vi "Adjust Focus.vi"(8 "error in":errorcluster, 10 "FocusPos":i64, 11 "Flir A700 in":refnum<class "Flir A700.lvclass">) -> (0 "error out":errorcluster, 3 "Flir A700 out":refnum<class "Flir A700.lvclass">)   [LabVIEW 2024, in "Flir A700.lvclass"]
uses:
  Flir A700.lvclass
  Flir A700.lvclass/Flir A700.ctl
  <resource>/objmgr/imaqdx.rc
  <vilib>/userDefined/High Color/IMAQdx.ctl
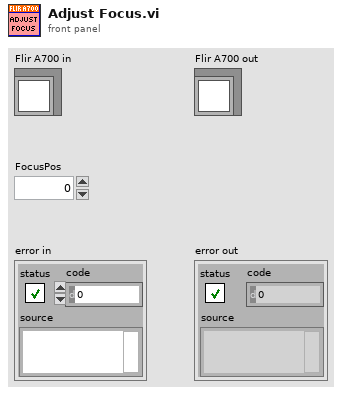
[diagram p1: front panel]
types:
  T1 = typedef "IMAQdx.ctl" = refnum<k21>
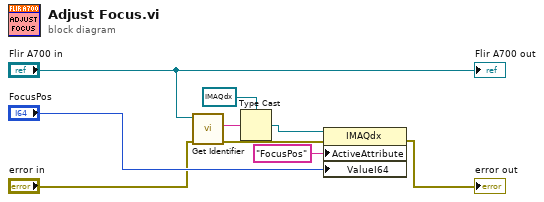
[diagram p0: block diagram]
diagram:
  n1 = call-dynamic "Get Identifier.vi"("Error In"="error in", "reference in"="Flir A700 in") -> ("Error Out"=w9:errorcluster, "Identifier"=w8:string)  [unwired: 7 in, 1 out]
  n2 = Type Cast(type=T1 refnum ("IMAQdx Session"), x=w8) -> (*(type *) &x=w6:T1)
  n3 = property class="IMAQdx"(reference=w6, error in=w9, "ActiveAttribute"="FocusPos", "ValueI64"="FocusPos") -> (error out=→"error out":errorcluster)  [unwired: 1 out]
  "Flir A700 out" <- "Flir A700 in"
